vi "CAN Daten sammeln.vi"(11 "Aktuelle Messwerte":sgl[](array[numeric])) -> ()   [LabVIEW 2020, in "Messdaten.lvlib"]
uses:
  Messdaten.lvlib
  Seiten/CAN Konfig/Aktion FGV CAN.ctl
  Seiten/CAN Konfig/CAN Konfig.lvlib
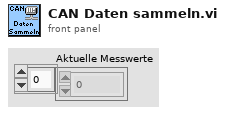
[diagram p1: front panel]
types:
  T1 = typedef "CAN Konfig.lvlib/Aktion FGV CAN.ctl" = enum16{"lesen", "schreiben Konfig", "Status", "Messdaten", "laden", "speichern", "CAN Data"}
  T2 = typedef "CAN Konfig.lvlib/CAN Messdaten.ctl" = cluster{"FTIR 1 Index":i32[], "FTIR 2 Index":i32[], "Status Index":i32[], "FT-IR Scale":sgl[], "Status Scale":sgl[], "Optionsfelder FT-IR":enum32{"Optionsauswahl 1", "Optionsauswahl 2", "Optionsauswahl 3"}, "Optionsfelder Status":enum32{"Optionsauswahl 1", "Optionsauswahl 2", "Optionsauswahl 3"}}
  T3 = enum32{"Optionsauswahl 1", "Optionsauswahl 2", "Optionsauswahl 3"}
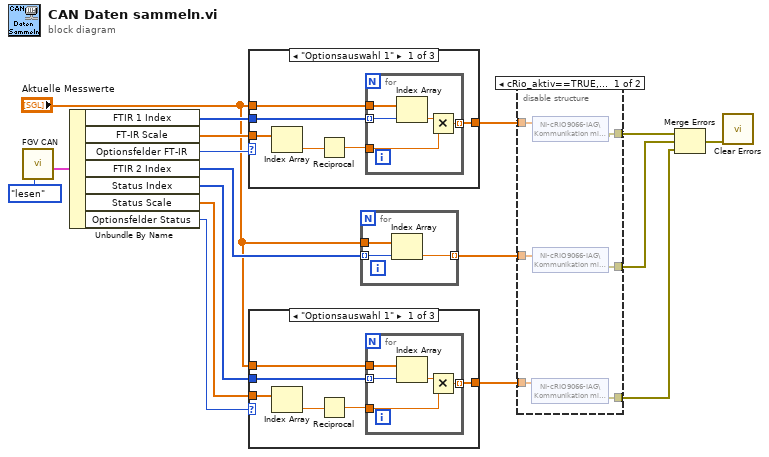
[diagram p0: block diagram]
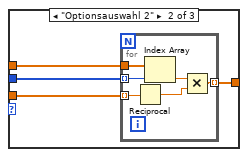
[diagram p3: hidden frame]
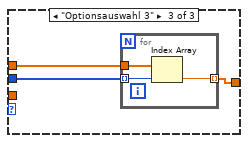
[diagram p4: hidden frame]
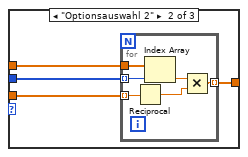
[diagram p5: hidden frame]
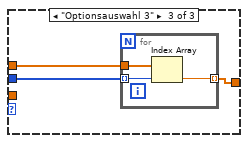
[diagram p6: hidden frame]
diagram:
  n1 = call "FGV CAN.vi"("Aktion"=Aktion_FGV_CAN."lesen") -> ("CAN Messdaten"=w9:T2)  [unwired: 6 in, 4 out]
  n2 = Unbundle By Name(w9) -> ("FTIR 1 Index"=w10:i32[], "FT-IR Scale"=w6:sgl[], "Optionsfelder FT-IR"=w7:T3, "FTIR 2 Index"=w11:i32[], "Status Index"=w3:i32[], "Status Scale"=w2:sgl[], "Optionsfelder Status"=w1:T3)
  n3 = case shown="\"Optionsauswahl 1\"" w7 {
    tunnel: [w23 w32 w41] -> w12
    tunnel: "Aktuelle Messwerte" -> [w22 w31 w40]
    tunnel: w10 -> [w21 w30 w39]
    tunnel: w6 -> [w20 w29 _]
    frame "Optionsauswahl 1" {
      n4 = Index Array(array=w20) -> (element=w19:sgl)  [unwired: 1 in]
      n5 = Reciprocal(x=w19) -> (1/x=w18:sgl)
      n6 = for {
        tunnel: w21 -> [w28] mode=indexing
        tunnel: w22 -> [w27]
        tunnel: [w25] -> w23 mode=indexing
        tunnel: w18 -> [w24]
        n7 = Index Array(array=w27, index=w28) -> (element=w26:sgl)
        n8 = Multiply(x=w26, y=w24) -> (x*y=w25:sgl)
      }
    }
    frame "Optionsauswahl 2" {
      n9 = for {
        tunnel: w30 -> [w38] mode=indexing
        tunnel: w31 -> [w37]
        tunnel: [w35] -> w32 mode=indexing
        tunnel: w29 -> [w34] mode=indexing
        n10 = Reciprocal(x=w34) -> (1/x=w33:sgl)
        n11 = Index Array(array=w37, index=w38) -> (element=w36:sgl)
        n12 = Multiply(x=w36, y=w33) -> (x*y=w35:sgl)
      }
    }
    frame "Optionsauswahl 3" {
      n13 = for {
        tunnel: w39 -> [w44] mode=indexing
        tunnel: w40 -> [w43]
        tunnel: [w42] -> w41 mode=indexing
        n14 = Index Array(array=w43, index=w44) -> (element=w42:sgl)
      }
    }
  }
  n15 = case shown="\"Optionsauswahl 1\"" w1 {
    tunnel: [w50 w59 w68] -> w5
    tunnel: "Aktuelle Messwerte" -> [w49 w58 w67]
    tunnel: w3 -> [w48 w57 w66]
    tunnel: w2 -> [w47 w56 _]
    frame "Optionsauswahl 1" {
      n16 = Index Array(array=w47) -> (element=w46:sgl)  [unwired: 1 in]
      n17 = Reciprocal(x=w46) -> (1/x=w45:sgl)
      n18 = for {
        tunnel: w48 -> [w55] mode=indexing
        tunnel: w49 -> [w54]
        tunnel: [w52] -> w50 mode=indexing
        tunnel: w45 -> [w51]
        n19 = Index Array(array=w54, index=w55) -> (element=w53:sgl)
        n20 = Multiply(x=w53, y=w51) -> (x*y=w52:sgl)
      }
    }
    frame "Optionsauswahl 2" {
      n21 = for {
        tunnel: w57 -> [w65] mode=indexing
        tunnel: w58 -> [w64]
        tunnel: [w62] -> w59 mode=indexing
        tunnel: w56 -> [w61] mode=indexing
        n22 = Reciprocal(x=w61) -> (1/x=w60:sgl)
        n23 = Index Array(array=w64, index=w65) -> (element=w63:sgl)
        n24 = Multiply(x=w63, y=w60) -> (x*y=w62:sgl)
      }
    }
    frame "Optionsauswahl 3" {
      n25 = for {
        tunnel: w66 -> [w71] mode=indexing
        tunnel: w67 -> [w70]
        tunnel: [w69] -> w68 mode=indexing
        n26 = Index Array(array=w70, index=w71) -> (element=w69:sgl)
      }
    }
  }
  n27 = for {
    tunnel: w11 -> [w74] mode=indexing
    tunnel: "Aktuelle Messwerte" -> [w73]
    tunnel: [w72] -> w13 mode=indexing
    n28 = Index Array(array=w73, index=w74) -> (element=w72:sgl)
  }
  n29 = disable-structure shown="cRio_aktiv==TRUE, Standard" {
    disable-tunnel: [w75 _] -> w16
    disable-tunnel: [w77 _] -> w15
    disable-tunnel: [w79 _] -> w14
    disable-tunnel: w13 -> [w78 _]
    disable-tunnel: w12 -> [w80 _]
    disable-tunnel: w5 -> [w76 _]
    frame condition #0 {
      n30 = shared-variable "NI-cRIO9066-IAG\\Kommunikation mit PC.lvlib\\Status"(w76) -> (error out=w75:errorcluster)  [unwired: 1 in]
      n31 = shared-variable "NI-cRIO9066-IAG\\Kommunikation mit PC.lvlib\\FTIR 1"(w80) -> (error out=w79:errorcluster)  [unwired: 1 in]
      n32 = shared-variable "NI-cRIO9066-IAG\\Kommunikation mit PC.lvlib\\FTIR 2"(w78) -> (error out=w77:errorcluster)  [unwired: 1 in]
    }
    frame condition #1 (active) {
    }
  }
  n33 = Merge Errors(w14, w15, w16) -> (w17:errorcluster)
  n34 = call <vilib>:"Clear Errors.vi"("error in (no error)"=w17) -> ()  [unwired: 5 in, 2 out]
